vi "File.Move File, Overwrite if Exists.vi"(8 "error in":errorcluster, 10 "Target Path":path, 11 "Source Path":path) -> (0 "error out":errorcluster, 3 "Target Out":path)   [LabVIEW 2024]
uses:
  Errors/Error.Error Code List.ctl
  Errors.lvlib
  <vilib>/KATE/Files/File Utils.lvlib
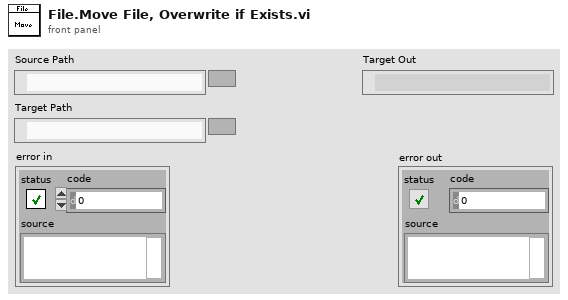
[diagram p1: front panel]
types:
  T1 = typedef "EQMF.lvlib/Errors.lvlib/Error.Error Code List.ctl" = i32
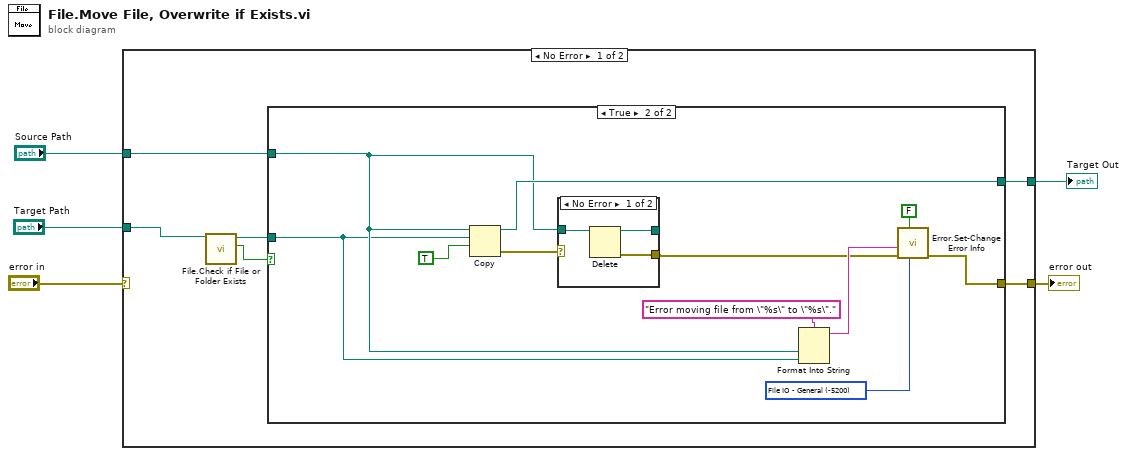
[diagram p0: block diagram]
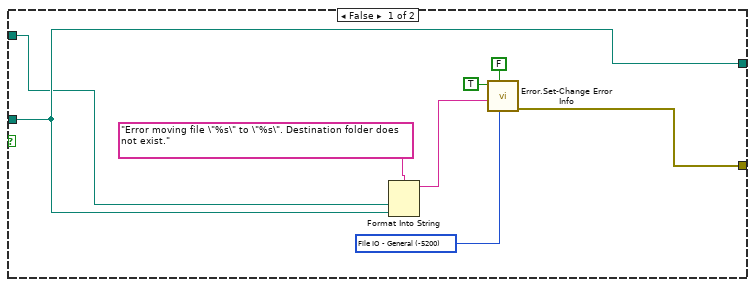
[diagram p2: hidden frame]
diagram:
  n1 = case shown="No Error" "error in" {
    selector: "error in" -> [_ w37]
    tunnel: "Target Path" -> [w8 w36]
    tunnel: [w9 w37] -> w4
    tunnel: "Source Path" -> [w10 _]
    tunnel: [w11 w36] -> w1
    frame No Error {
      n2 = call <vilib>:"File.Check if File or Folder Exists.vi"("Path"=w8) -> ("Exists"=w6:bool, "Dup Path"=w7:path)  [unwired: 6 in, 3 out]
      n3 = case shown="True" w6 {
        tunnel: [w13 w30] -> w11
        tunnel: w10 -> [w12 w25]
        tunnel: [w15 w23] -> w9
        tunnel: w7 -> [w13 w20]
        frame False {
          w17 = T1 -5200 items=["No Error"=0, "Abort"=-2, "Misc"=-5000, "Fixture Error"=-5100, "File IO - General"=-5200, "FIle IO - Config Error"=-5201, "Instrument - General"=-5300, "Instrument - Serial Com"=-5301, "Instrument - Camera"=-5302, "Instrument - PS"=-5303, "Instrument - Oscilloscope"=-5304, "Instrument - Function Gen"=-5305, "Instrument - Load"=-5306, "Instrument - Meter"=-5307, "Instrument - Power Control"=-5308, "Instrument - Motion"=-5309, "Instrument - RF"=-5310, "System Exe"=-5400, "Image Processing"=-5500, "Communication"=-5600, "Script - Syntax Error"=-6000, "Script - Invalid Name or Param"=-6100, "Script - Timeout"=-6200, "Invalid Data"=-6300, "FW Update Error"=-6500] ("Std Code")
          n4 = Format Into String(format string="Error moving file \"%s\" to \"%s\". Destination folder does not exist.", w12, w13) -> (resulting string=w18:string)  [unwired: 2 in, 1 out]
          n5 = call "Error.Set-Change Error Info.vi"("Std Code"=w17, "Append Details"=FALSE, "Description"=w18, "Set Error"=TRUE) -> ("error out"=w15:errorcluster)  [unwired: 7 in]
        }
        frame True {
          w24 = T1 -5200 items=["No Error"=0, "Abort"=-2, "Misc"=-5000, "Fixture Error"=-5100, "File IO - General"=-5200, "FIle IO - Config Error"=-5201, "Instrument - General"=-5300, "Instrument - Serial Com"=-5301, "Instrument - Camera"=-5302, "Instrument - PS"=-5303, "Instrument - Oscilloscope"=-5304, "Instrument - Function Gen"=-5305, "Instrument - Load"=-5306, "Instrument - Meter"=-5307, "Instrument - Power Control"=-5308, "Instrument - Motion"=-5309, "Instrument - RF"=-5310, "System Exe"=-5400, "Image Processing"=-5500, "Communication"=-5600, "Script - Syntax Error"=-6000, "Script - Invalid Name or Param"=-6100, "Script - Timeout"=-6200, "Invalid Data"=-6300, "FW Update Error"=-6500] ("Std Code")
          n6 = Copy(9:TRUE ("overwrite (F)"), 10:w20, 11:w25) -> (0:w29:errorcluster, 3:w30:path)  [unwired: 2 in, 1 out]
          n7 = case shown="No Error" w29 {
            selector: w29 -> [_ w34]
            tunnel: w25 -> [w33 w35]
            tunnel: [w32 w34] -> w26
            tunnel: [w31 w35] -> _
            frame No Error {
              n8 = Delete(path (use dialog)=w33) -> (deleted path=w31:path, error out=w32:errorcluster)  [unwired: 4 in, 1 out]
            }
            frame Error {
            }
          }
          n9 = Format Into String(format string="Error moving file from \"%s\" to \"%s\".", w25, w20) -> (resulting string=w27:string)  [unwired: 2 in, 1 out]
          n10 = call "Error.Set-Change Error Info.vi"("Std Code"=w24, "Append Details"=FALSE, "error in"=w26, "Description"=w27) -> ("error out"=w23:errorcluster)  [unwired: 7 in]
        }
      }
    }
    frame Error {
    }
  }
  "error out" <- w4
  "Target Out" <- w1
